vi "Measure distance v2.vi"(8 "error in (no error)":errorcluster, 11 "Input image":T3=refnum) -> (0 "error out":errorcluster)   [LabVIEW 2020]
uses:
  <vilib>/vision/Image Controls.llb/IMAQ Image.ctl
  OOP/MulColLBTable/Object operations.ctl
  Globals/Event FGV Actions.ctl
  TypeDefs/data and image buffer fgv actions.ctl
  <vilib>/Utility/error.llb/whitespace.ctl
  <vilib>/vision/NI_Vision_Development_Module.lvlib
  OOP/MulColLBTable/MulColLBTable-Array/MulColLBTable-Array.lvclass
panel:
  in  "Tab Control":T1(tab)
  in  "Distinct Colours":bool
  in  "Overlay Selected":bool
  in  "Overlay All":bool
  in  "Remove Selected":bool
  in  "Image buffer - Imaging Parameters":i32[](listbox)
  in  "Image buffer - Calibration Parameters":i32[](listbox)
  out "Array 2":dbl[](array[numeric])
  out "min value":dbl
  out "Array":cdb[](array[numeric])
  out "Coordinates":i32[](array[numeric])
  out "Distances":dbl[][](array[numeric])
  out "error out 5":errorcluster
  out "error out 3":errorcluster
  out "error out 7":errorcluster
  out "error out 6":errorcluster
  out "error out 4":errorcluster
  out "Last Mouse Position:All Elements":cluster{"X":i32, "Y":i32}
  out "Circles Data":T2(array[cluster])
  in  "Min Radius":sgl=3.0
  in  "Max Radius":sgl=100.0
  in  "Number of iterations (1)":i32=1
  out "Minimal Value":sgl
  out "Maximal Value":sgl
  out "Image Pixels (U8)":u8[][](array[numeric])
  out "Image size changed":bool
  out "error out 8":errorcluster
  out "error out 9":errorcluster
  out "error out 11":errorcluster
  out "error out 10":errorcluster
  out "Distances 2":sgl[](array[numeric]) format="%.4f"
  in  "Clear Images":bool
  in  "Clear Measurements":bool
  in  "Measurement Mode":T4(ring)
  in  "Re-instate":bool
  out "output cluster":T5 {"Y" format="%.2f"; "X" format="%.2f"}
  out "Image Pixels (I16) 2":i16[][](array[numeric])
  in  "Tab Control 2":enum32{"Grayscale", "Binary", "Intensity"}(tab)
  in  "All":bool
  out "Output Image":T3(plugin-control)
  in  "Grid":bool
  in  "Grid Lines":u32=2 min=1 max=100 step=1
  in  "Image Selector":i32(c297)=7
  out "Output Image 2":T3(plugin-control)
  out "Intensity Graph":i16[][](graph)
  in  "Operation":T6(ring)
  in  "Vertical Pointer Slide":cluster{"Numeric":dbl, "Numeric":dbl}(slide)={"Numeric"=0.0, "Numeric"=254.0} scale=0.0..4096.0
  in  "stop":bool
  # "X Start"
  # "Y start"
  # "X Stop"
  # "X Dist"
  # "Dist"
  # "Y Stop"
  # "Y Dist"
  # "PROTOTYPE ONLY"
  # "This utility is under development, please report any \nissues to the contact details provided on github"
  # "Note : Closing the VI using the top right window close ('X') will only close the front panel - VI keeps running.\nTo completely close this window click 'FINISH/EXIT'"
  # "Current Image data"
  # "Image Processing routines"
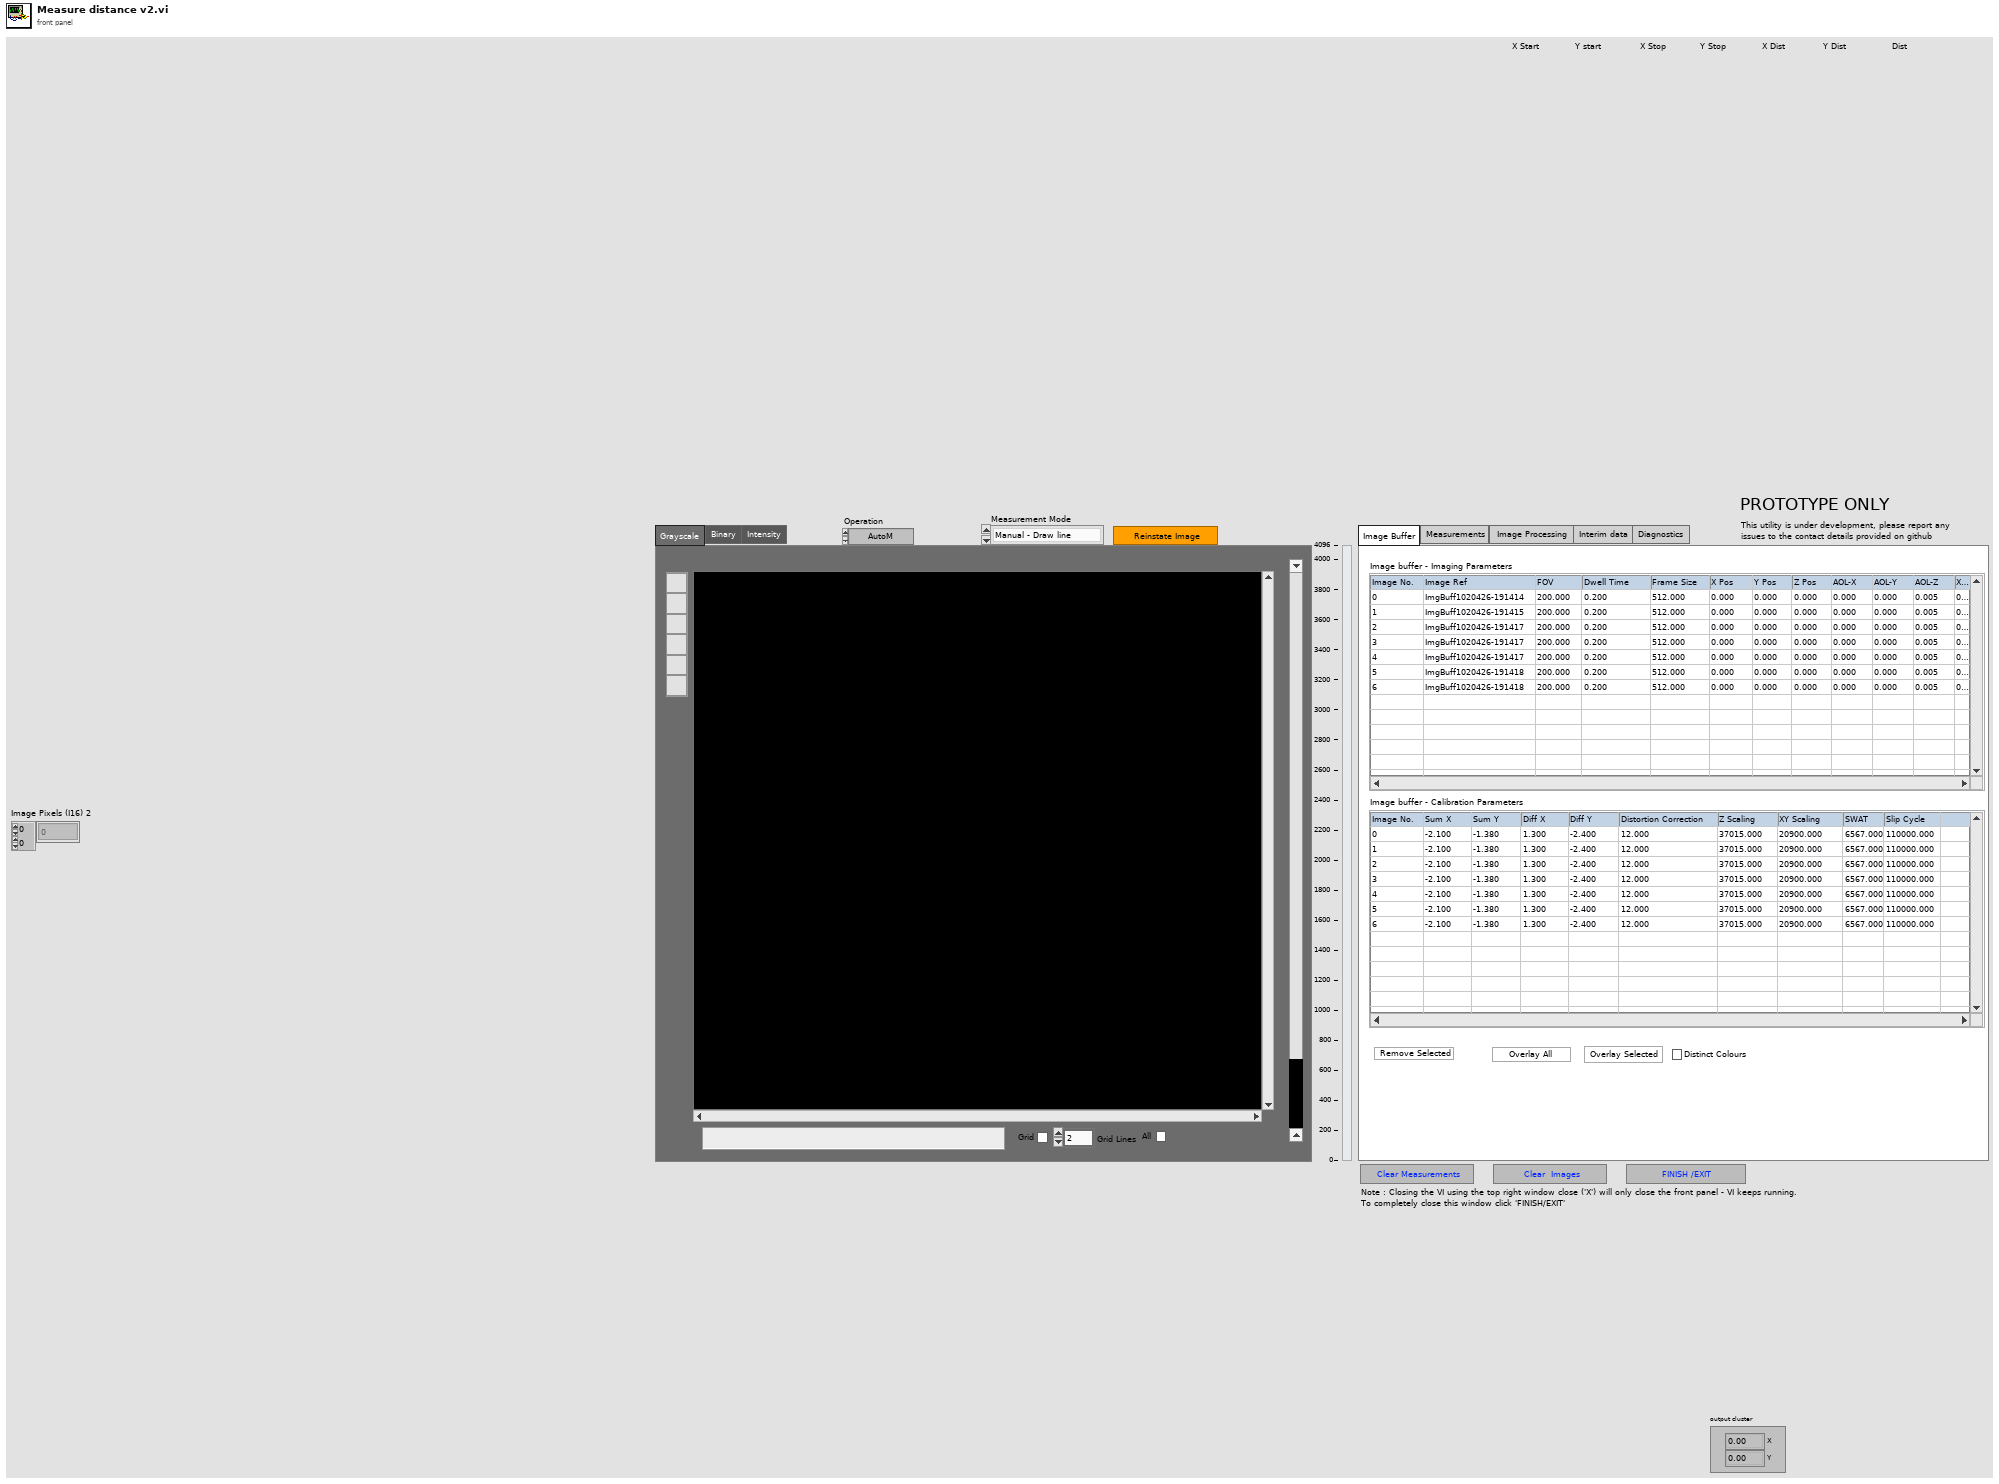
[diagram p1: front panel]
types:
  T1 = enum32{"Image Buffer", "Measurements", "Image Processing  ", "Interim data", "Diagnostics"}
  T2 = cluster{"Pos. X":i32, "Pos. Y":i32, "Radius":i32, "Core Area":i32}[]
  T3 = typedef "IMAQ Image.ctl" = refnum<image>
  T4 = enum16{"Manual - Draw line", "Manual - Circles", "Manual - Points", "Automatic - Circles", "Automatic - Points"}
  T5 = typedef "IMAQ Point" = cluster{"X":sgl, "Y":sgl}
  T6 = enum32{"AutoM", "Close", "Dilate", "Erode", "Gradient", "Gradient out", "Gradient in", "Hit miss", "Open", "PClose", "POpen", "Thick", "Thin"}
  T7 = typedef "Event FGV Actions.ctl" = enum16{"Register Event", "Fire Event", "Release Event"}
  T8 = typedef "Object operations.ctl" = enum16{"Initialise", "Add column headers", "Add rows - bulk", "Stack row - single", "Stack row - multi", "Select row(s)", "Delete row(s)", "Destroy"}
  T9 = typedef "ROI Descriptor" = cluster{"Global Rectangle":i32[], "Contours":cluster{"ID":enum32{"External", "Internal"}, "Type":u32, "Coordinates":i32[]}[]}
  T10 = typedef "data and image buffer fgv actions.ctl" = enum16{"Initialise", "Add Image to buffer", "Read Image buffer", "Edit specific data", "Delete selected image", "Clear all images"}
  T11 = typedef "IMAQ Circle" = cluster{"Center X":i32, "Center Y":i32, "Inner Radius":i32, "Outer Radius":i32, "Start Angle":dbl, "End Angle":dbl}
  T12 = typedef "Current Imaging Parameters.ctl" = cluster{"FOV":dbl, "Dwell Time":dbl, "Frame Size":dbl, "XPos":dbl, "YPos":dbl, "ZPos":dbl, "AOL-X":dbl, "AOL-Y":dbl, "AOL-Z":dbl, "X-Angle":dbl, "Y-Angle":dbl, "Z-Angle":dbl}
  T13 = typedef "Current Calibration Parameters.ctl" = cluster{"Sum X":dbl, "Sum Y":dbl, "Diff X":dbl, "Diff Y":dbl, "Distortion Correction":dbl, "Z_norm to um_scaling":dbl, "X_norm to um_scaling":dbl, "Samples to Wait after Trigger":dbl, "Slip Cycle":dbl}
  T14 = typedef "Image Type" = u32
  T15 = cluster{"histogram":u32[], "Minimal Value":sgl, "Maximal Value":sgl, "Starting Value":sgl, "Interval Width":sgl, "Mean Value":sgl, "Standard  Variation":sgl, "Area (pixels)":i32}
  T16 = typedef "IMAQ Line" = cluster{"Start X":i32, "Start Y":i32, "End X":i32, "End Y":i32}
  T17 = cluster{"Pos. X":i32, "Pos. Y":i32, "Radius":i32, "Core Area":i32}
  T18 = typedef "whitespace.ctl" = u16
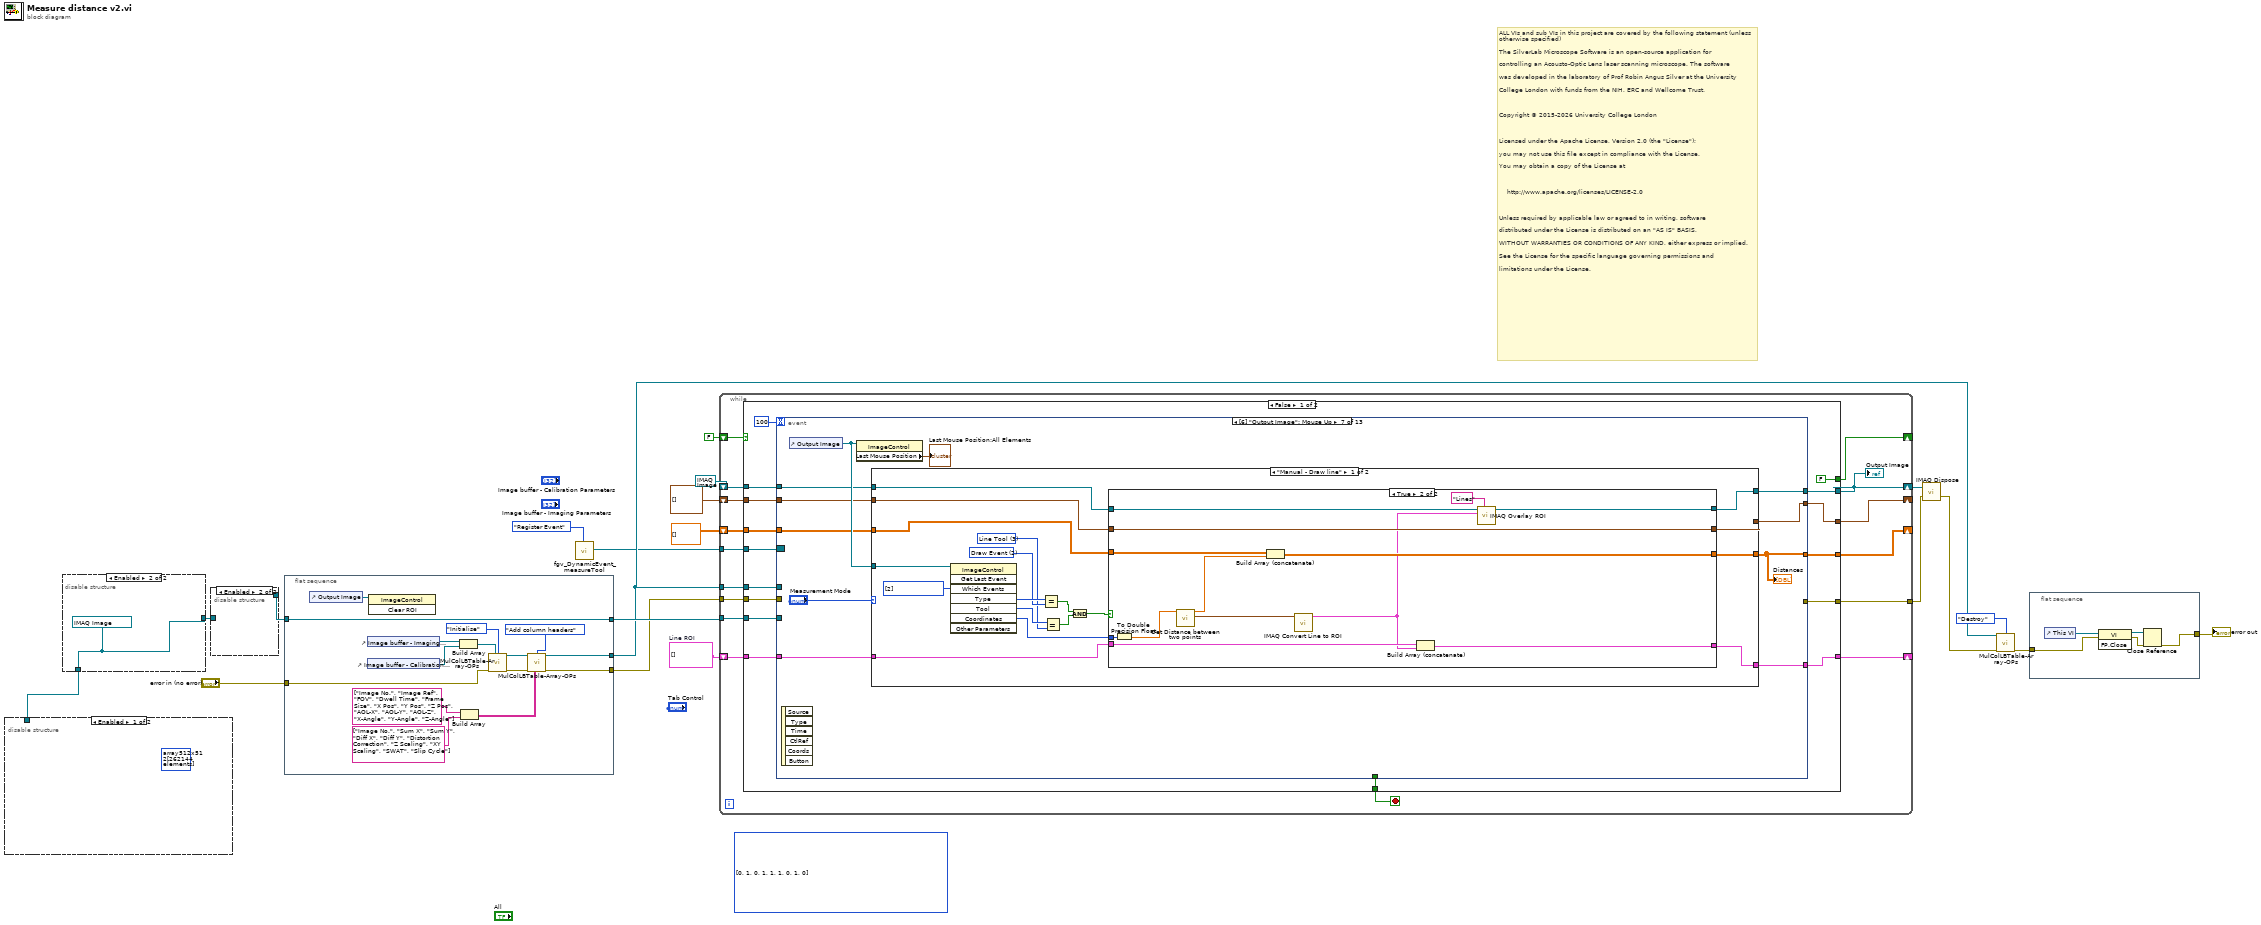
[diagram p0: block diagram]
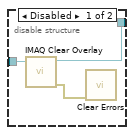
[diagram p2: hidden frame]
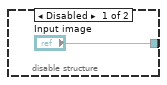
[diagram p3: hidden frame]
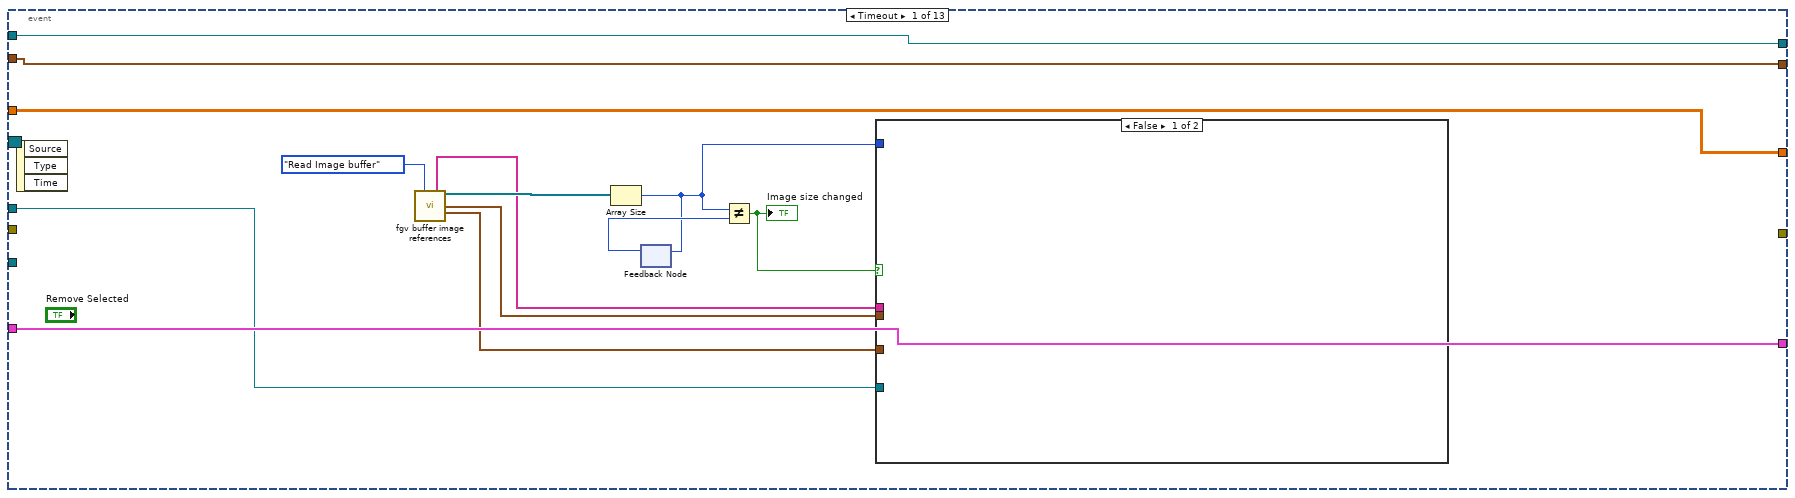
[diagram p5: hidden frame]
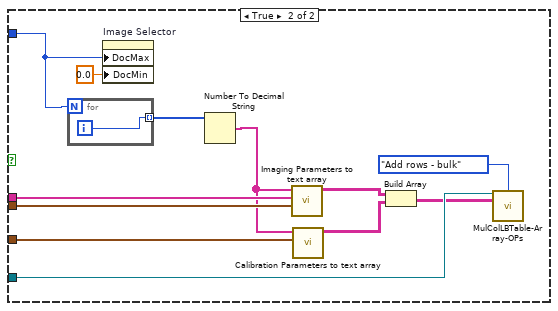
[diagram p6: hidden frame]
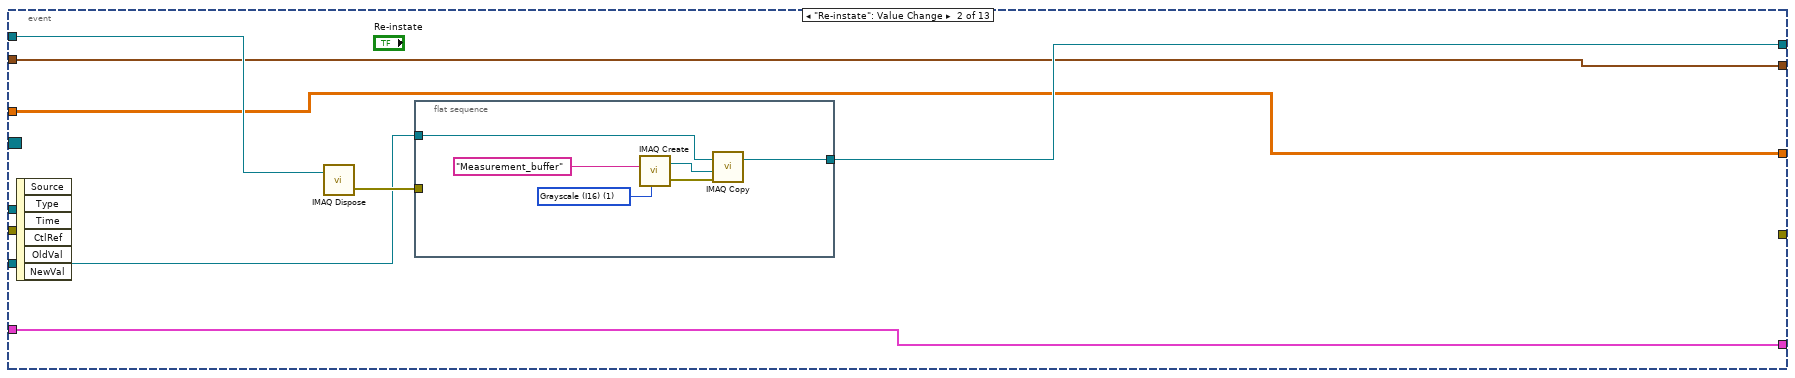
[diagram p7: hidden frame]
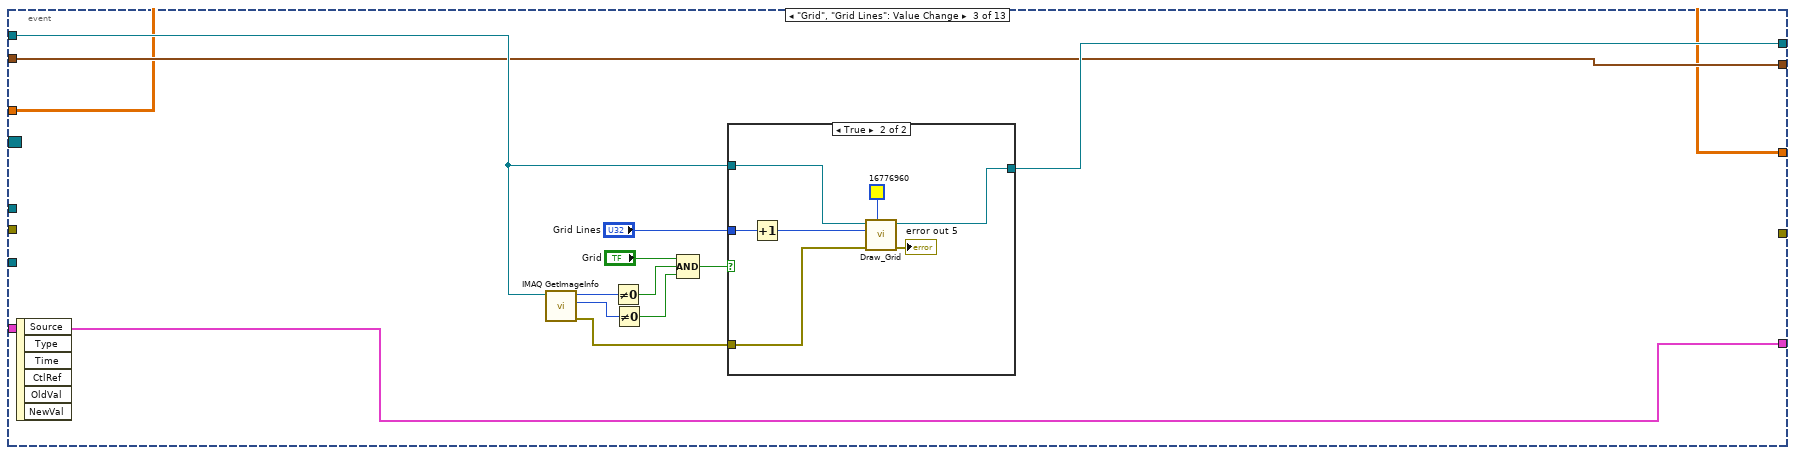
[diagram p8: hidden frame]
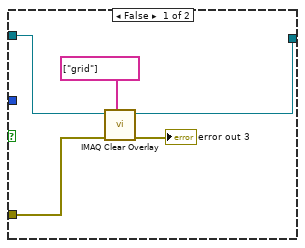
[diagram p9: hidden frame]
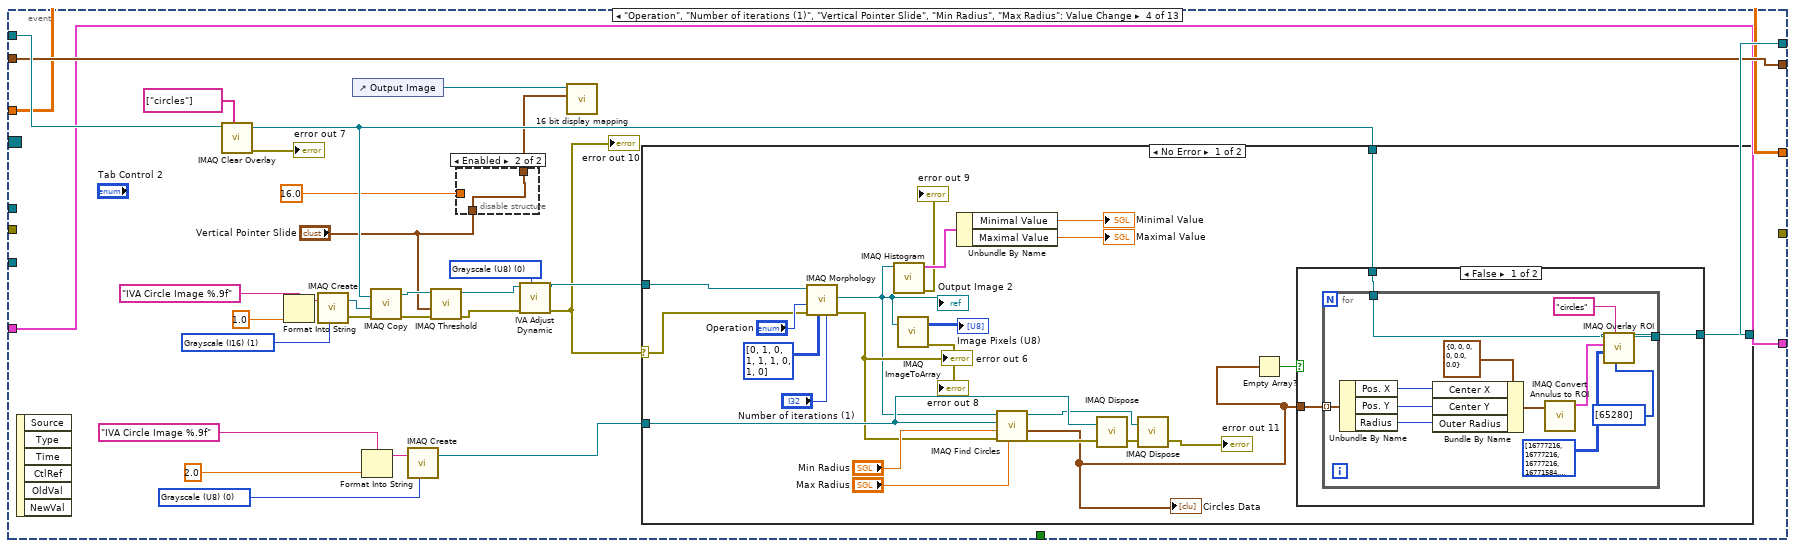
[diagram p10: hidden frame]
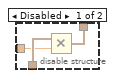
[diagram p11: hidden frame]
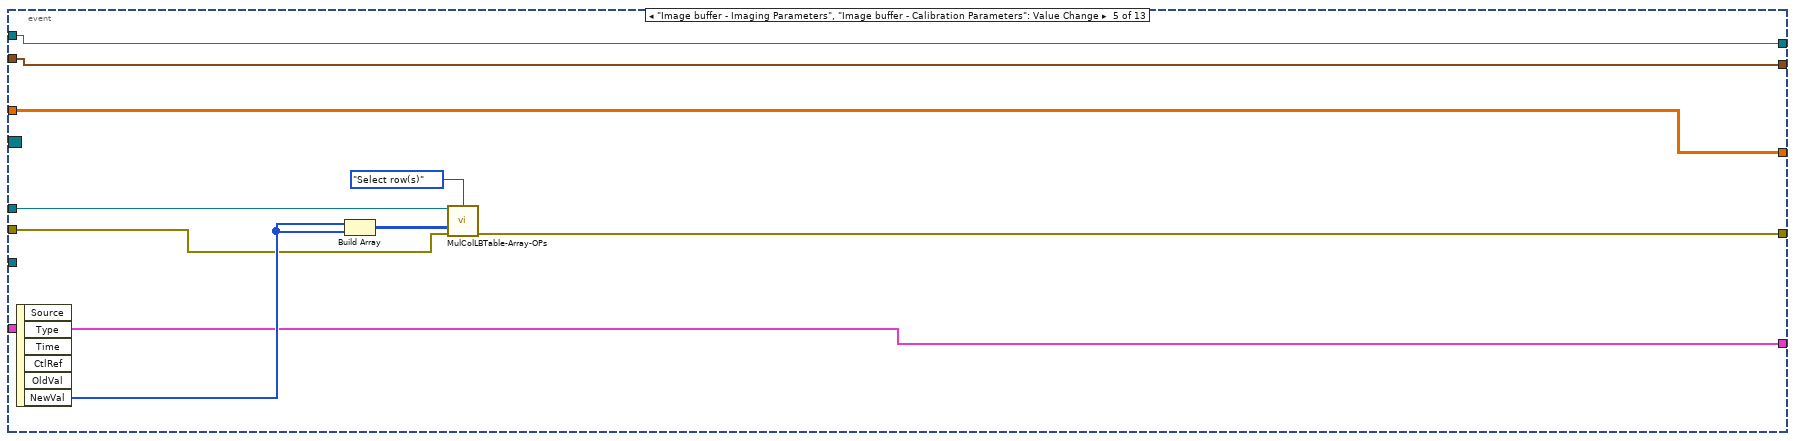
[diagram p14: hidden frame]
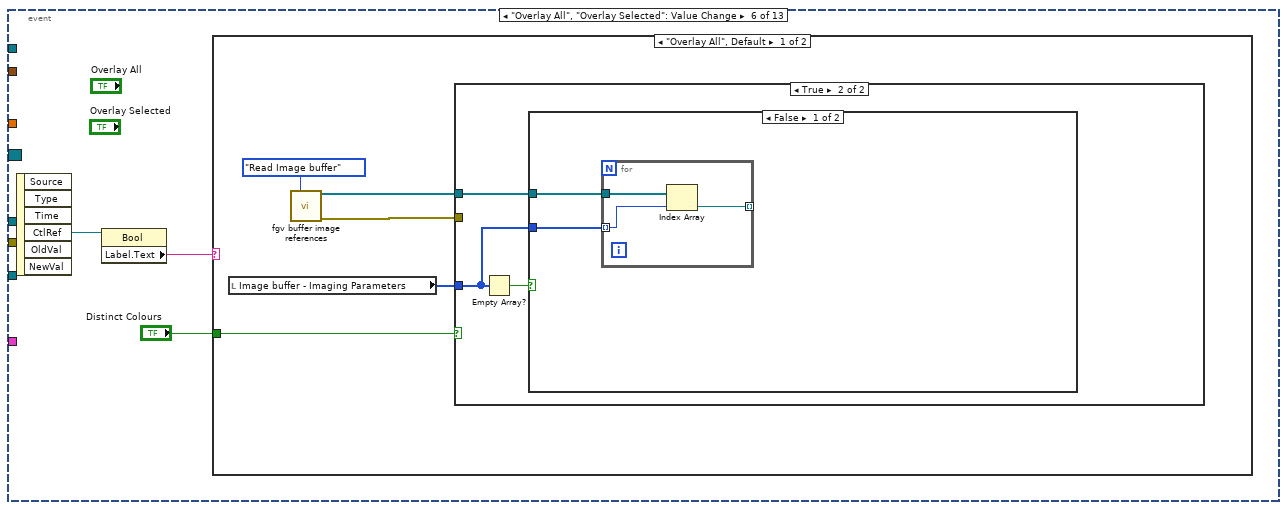
[diagram p15: hidden frame]
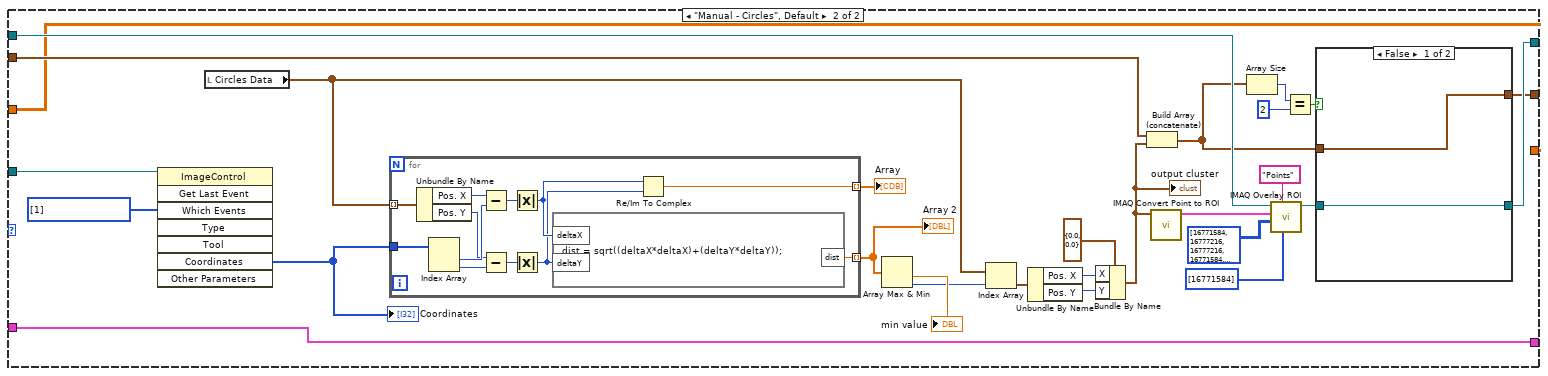
[diagram p20: hidden frame]
diagram:
  w15 = T9[] []  # Line ROI
  (unwired) i32[][] [[0, 1, 0], [1, 1, 1], [0, 1, 0]] ("Structuring Element (Basic Morphology 1) 2")
  # "ALL VIs and sub VIs in this project are covered by the following statement (unless \notherwise specified)\n\nThe SilverLab Microscope Software is an open-source application for\n\ncontrolling an Acousto-Optic Lens laser scanning microscope. The software\n\nwas developed in the laboratory of Prof Robin Angus Silver at the University\n\nCollege London with funds from the NIH, ERC and Wellcome Trust.\n\n \n\nCopyright © 2015-2026 University College London\n\n \n\nLicensed under the Apache License, Version 2.0 (the \"License\");\n\nyou may not use this file except in compliance with the License.\n\nYou may obtain a copy of the License at\n\n \n\n    http://www.apache.org/licenses/LICENSE-2.0\n\n \n\nUnless required by applicable law or agreed to in writing, software\n\ndistributed under the License is distributed on an \"AS IS\" BASIS,\n\nWITHOUT WARRANTIES OR CONDITIONS OF ANY KIND, either express or implied.\n\nSee the License for the specific language governing permissions and\n\nlimitations under the License."
  n1 = disable-structure shown="Enabled" {
    disable-tunnel: ["Input image" w22] -> w14
    disable-tunnel: [_ w22] -> w18
    frame Disabled {
    }
    frame Enabled {
      w22 = T3 refnum ("Input image 2")
    }
  }
  n2 = disable-structure shown="Enabled" {
    disable-tunnel: w18 -> [_ _]
    frame Enabled {
      (unwired) i16[][] array512x512[262144 elements] ("Image Pixels (I16) 2")
    }
    frame Disabled {
    }
  }
  n3 = disable-structure shown="Enabled" {
    disable-tunnel: w14 -> [w25 _]
    disable-tunnel: [w23 _] -> w13
    frame Disabled {
      n4 = call "IMAQ Clear Overlay"("Image"=w25) -> ("error out"=w24:errorcluster, "Image Out"=w23:T3)  [unwired: 9 in]
      n5 = call <vilib>:"Clear Errors.vi"("error in (no error)"=w24) -> ()  [unwired: 5 in, 2 out]
    }
    frame Enabled {
    }
  }
  n6 = flat-sequence {
    tunnel: w13 -> [w39]
    tunnel: [w39] -> w12
    tunnel: [w28] -> w9
    tunnel: [w27] -> w10
    tunnel: "error in (no error)" -> [w26]
    frame #0 {
      n7 = control-ref of="Output Image"() -> (w40:refnum<vi>)
      n8 = control-ref of="Image buffer - Imaging Parameters"() -> (w37:refnum<vi>)
      n9 = control-ref of="Image buffer - Calibration Parameters"() -> (w38:refnum<vi>)
      n10 = invoke class="ImageControl" method="Clear ROI"(reference=w40) -> ()  [unwired: 2 in, 3 out]
      n11 = Build Array(w37, w38) -> (w36:refnum<vi>[])
      n12 = Build Array(string[] ["Image No.", "Image Ref", "FOV", "Dwell Time", "Frame Size", "X Pos", "Y Pos", "Z Pos", "AOL-X", "AOL-Y", "AOL-Z", "X-Angle", "Y-Angle", "Z-Angle"] ("Column Header Strings[]"), string[] ["Image No.", "Sum X", "Sum Y", "Diff X", "Diff Y", "Distortion Correction", "Z Scaling", "XY Scaling", "SWAT", "Slip Cycle"] ("Column Header Strings[]")) -> (w29:string[][])
      n13 = call "MulColLBTable-Array-OPs.vi"("Multi-col LB Refs"=w36, "Operations"=Object_operations."Initialise", "error in (no error)"=w26) -> ("MulColLBTable-Array.lvclass OUT"=w33:refnum<class "MulColLBTable-Array.lvclass">, "error out"=w34:errorcluster)  [unwired: 11 in]
      n14 = call "MulColLBTable-Array-OPs.vi"("MulColLBTable-Array.lvclass IN"=w33, "Operations"=Object_operations."Add column headers", "error in (no error)"=w34, "Column Header Strings[]"=w29) -> ("MulColLBTable-Array.lvclass OUT"=w28:refnum<class "MulColLBTable-Array.lvclass">, "error out"=w27:errorcluster)  [unwired: 10 in]
    }
  }
  n15 = call "fgv_DynamicEvent_measureTool.vi"("Event FGV Actions"=Event_FGV_Actions."Register Event") -> ("Event Registration Refnum"=w3:refnum<event-registration>)  [unwired: 8 in, 2 out]
  n16 = while {
    shift-right: [w52] -> _
    shift-left: FALSE -> [w56]
    tunnel: w12 -> [w55]
    shift-right: [w51] -> w17
    shift-left: T3 refnum ("Image Dst Out") -> [w54]
    shift-right: [w49] -> _
    shift-left: T5[] [] -> [w50]
    shift-right: [w47] -> _
    shift-left: dbl[][] [] ("Distances 2") -> [w48]
    shift-right: [w45] -> _
    shift-left: w15 -> [w46]
    tunnel: w9 -> [w44]
    tunnel: w10 -> [w43]
    tunnel: [w42] -> w5
    tunnel: w3 -> [w41]
    stop <- w53 stop-if-true
    n17 = case shown="False" w56 {
      tunnel: w55 -> [w65 w384]
      tunnel: [w71 w382] -> w51
      tunnel: w54 -> [w72 _]
      tunnel: [w69 FALSE] -> w53
      tunnel: [FALSE FALSE] -> w52
      tunnel: w50 -> [w67 w381]
      tunnel: [w66 w381] -> w49
      tunnel: w48 -> [w64 w379]
      tunnel: [w63 w379] -> w47
      tunnel: w46 -> [w62 w378]
      tunnel: [w61 w378] -> w45
      tunnel: w44 -> [w60 _]
      tunnel: w43 -> [w59 _]
      tunnel: [w58 _] -> w42
      tunnel: w41 -> [w57 _]
      frame False {
        n18 = event shown="[6] \"Output Image\": Mouse Up" {
          selector: w57 -> [_ _ _ _ _ _ _ _ _ _ _ _ _]
          dyn-events: _ -> [_ _ _ _ _ _ _ _ _ _ _ _ _]
          timeout: 100 -> [_ _ _ _ _ _ _ _ _ _ _ _ _]
          tunnel: w72 -> [w85 w105 w123 w152 w216 _ w246 w338 w346 _ _ w364 w375]
          tunnel: [w85 w102 w124 w154 w216 _ w245 w336 w346 w348 _ w364 w375] -> w71
          tunnel: [_ _ _ _ _ _ _ _ _ _ FALSE TRUE w366] -> w69
          tunnel: w67 -> [w84 w101 w114 w149 w215 _ w243 w339 w345 w356 _ w363 w374]
          tunnel: [w84 w101 w114 w149 w215 _ w244 w339 w345 w356 _ w363 w374] -> w66
          tunnel: w65 -> [_ w103 _ _ _ _ _ _ _ _ _ _ _]
          tunnel: w64 -> [w83 w99 w113 w145 w214 _ w241 _ w344 w355 _ w362 w373]
          tunnel: [w83 w99 w113 w145 w214 _ w238 w341 w344 w355 _ w362 w373] -> w63
          tunnel: w62 -> [w82 w100 w112 w144 w212 _ w240 _ w343 w354 _ w361 w372]
          tunnel: [w82 w100 w112 w144 w212 _ w239 w340 w343 w354 _ w361 w372] -> w61
          tunnel: w60 -> [w74 _ _ _ w221 _ _ _ _ _ _ _ _]
          tunnel: w59 -> [_ _ _ _ w217 _ _ _ _ _ _ _ _]
          tunnel: [_ _ _ _ w213 _ _ _ _ _ _ _ _] -> w58
          event Timeout {
            n19 = event-data() -> ()  [unwired: 1 in, 3 out]
            n20 = call "fgv buffer image references.vi"("Actions"=data_and_image_buffer_fgv_actions."Read Image buffer") -> ("Imag ref. name"=w75:string[], "Image Array"=w76:T3[], "Imaging Parameters"=w78:T12[], "Calibration Parameters"=w77:T13[])  [unwired: 8 in, 3 out]
            n21 = Array Size(array=w76) -> (size(s)=w79:i32)
            n22 = feedback-in #1(w79) -> ()
            n23 = feedback #1() -> (w81:i32)  [unwired: 1 in]
            n24 = Not Equal?(x=w79, y=w81) -> (x != y?=w80:bool)
            "Image size changed" <- w80
            n25 = case shown="False" w80 {
              tunnel: w79 -> [_ w95]
              tunnel: w78 -> [_ w93]
              tunnel: w77 -> [_ w91]
              tunnel: w75 -> [_ w94]
              tunnel: w74 -> [_ w88]
              frame False {
              }
              frame True {
                n26 = for {
                  N: w95 -> [_]
                  tunnel: [w98] -> w96 mode=indexing
                  i -> [w98]
                }
                n27 = property on="Image Selector" class="Scroll (strict)"("DocMax"=w95, "DocMin"=0.0 ("Doc Min")) -> ()  [unwired: 2 in, 2 out]
                n28 = Number To Decimal String(number=w96) -> (decimal integer string=w92:string[])  [unwired: 1 in]
                n29 = call "Imaging Parameters to text array.vi"("Imaging Parameters"=w93, "Image Ref"=w94, "Image No"=w92) -> ("Imaging Parameters"=w90:string[][])  [unwired: 8 in]
                n30 = call "Calibration Parameters to text array.vi"("Calibration Parameters"=w91, "Image No"=w92) -> ("Calibration Parameters"=w89:string[][])  [unwired: 9 in]
                n31 = Build Array(w90, w89) -> (w86:string[][][])
                n32 = call "MulColLBTable-Array-OPs.vi"("MulColLBTable-Array.lvclass IN"=w88, "Operations"=Object_operations."Add rows - bulk", "Item Names - Bulk / stack Multiple"=w86) -> ()  [unwired: 11 in, 2 out]
              }
            }
          }
          event "Re-instate": Value Change {
            n33 = event-data() -> ()  [unwired: 1 in, 6 out]
            n34 = call "IMAQ Dispose"("Image"=w105) -> ("error out"=w104:errorcluster)  [unwired: 5 in]
            n35 = flat-sequence {
              tunnel: w104 -> [_]
              tunnel: w103 -> [w107]
              tunnel: [w106] -> w102
              frame #0 {
                w108 = T14 1 items=["Grayscale (U8)", "Grayscale (I16)", "Grayscale (SGL)", "Complex (CSG)", "RGB (U32)", "HSL (U32)", "RGB (U64)", "Grayscale (U16)"] ("Image Type")
                n36 = call "IMAQ Create"("Image Name"="Measurement_buffer", "Image Type"=w108) -> ("New Image"=w110:T3, "error out"=w111:errorcluster)  [unwired: 3 in]
                n37 = call "IMAQ Copy"("error in (no error)"=w111, "Image Dst"=w110, "Image Src"=w107) -> ("Image Dst Out"=w106:T3)  [unwired: 3 in, 1 out]
              }
            }
          }
          event "Grid", "Grid Lines": Value Change {
            n38 = event-data() -> ()  [unwired: 1 in, 6 out]
            n39 = call "IMAQ GetImageInfo"("Image"=w123) -> ("error out"=w117:errorcluster, "Y Resolution"=w120:i32, "X Resolution"=w121:i32)  [unwired: 3 in, 5 out]
            n40 = Not Equal To 0?(x=w121) -> (x != 0?=w119:bool)
            n41 = Not Equal To 0?(x=w120) -> (x != 0?=w118:bool)
            n42 = Compound Arithmetic op=AND("Grid", w119, w118) -> (w116:bool)
            n43 = case shown="True" w116 {
              tunnel: w123 -> [w128 w136]
              tunnel: [w127 w135] -> w124
              tunnel: w117 -> [w125 w133]
              tunnel: "Grid Lines" -> [_ w131]
              frame False {
                n44 = call "IMAQ Clear Overlay"("Groups"=string[] ["grid"], "error in (no error)"=w125, "Image"=w128) -> ("error out"=→"error out 3":errorcluster, "Image Out"=w127:T3)  [unwired: 7 in]
              }
              frame True {
                n45 = Increment(x=w131) -> (x+1=w130:u32)
                n46 = call "Draw_Grid.vi"("Grid Line Color"=u32 16776960, "error in (no error)"=w133, "Grid Lines"=w130, "Image In"=w136) -> ("error out"=→"error out 5":errorcluster, "Image Out"=w135:T3)  [unwired: 6 in]
              }
            }
          }
          event "Operation", "Number of iterations (1)", "Vertical Pointer Slide", "Min Radius", "Max Radius": Value Change {
            w158 = T14 0 items=["Grayscale (U8)", "Grayscale (I16)", "Grayscale (SGL)", "Complex (CSG)", "RGB (U32)", "HSL (U32)", "RGB (U64)", "Grayscale (U16)"] ("Image Type")
            w159 = T14 0 items=["Grayscale (U8)", "Grayscale (I16)", "Grayscale (SGL)", "Complex (CSG)", "RGB (U32)", "HSL (U32)", "RGB (U64)", "Grayscale (U16)"] ("Image Type")
            w164 = T14 1 items=["Grayscale (U8)", "Grayscale (I16)", "Grayscale (SGL)", "Complex (CSG)", "RGB (U32)", "HSL (U32)", "RGB (U64)", "Grayscale (U16)"] ("Image Type")
            n47 = event-data() -> ()  [unwired: 1 in, 6 out]
            n48 = call "IMAQ Clear Overlay"("Groups"=string[] ["circles"], "Image"=w152) -> ("error out"=→"error out 7":errorcluster, "Image Out"=w151:T3)  [unwired: 8 in]
            n49 = Format Into String(format string="IVA Circle Image %.9f" ("Image Name"), 1.0) -> (resulting string=w166:string)  [unwired: 2 in, 1 out]
            n50 = call "IMAQ Create"("Image Name"=w166, "Image Type"=w164) -> ("New Image"=w156:T3, "error out"=w157:errorcluster)  [unwired: 2 in, 1 out]
            n51 = control-ref of="Output Image"() -> (w148:refnum<vi>)
            n52 = Format Into String(format string="IVA Circle Image %.9f" ("Image Name"), 2.0) -> (resulting string=w162:string)  [unwired: 2 in, 1 out]
            n53 = call "IMAQ Copy"("error in (no error)"=w157, "Image Dst"=w156, "Image Src"=w151) -> ("error out"=w142:errorcluster, "Image Dst Out"=w143:T3)  [unwired: 3 in]
            n54 = call "IMAQ Create"("Image Name"=w162, "Image Type"=w159) -> ("New Image"=w155:T3)  [unwired: 2 in, 2 out]
            n55 = call "IMAQ Threshold"("error in (no error)"=w142, "Range"="Vertical Pointer Slide", "Image Src"=w143) -> ("error out"=w141:errorcluster, "Image Dst Out"=w140:T3)  [unwired: 3 in, 4 out]
            n56 = disable-structure shown="Enabled" {
              disable-tunnel: "Vertical Pointer Slide" -> [w169 w170]
              disable-tunnel: 16.0 -> [w168 _]
              disable-tunnel: [w167 w170] -> w146
              frame Disabled {
                n57 = Multiply(x=w169, y=w168) -> (x*y=w167:cluster{"Numeric":dbl, "Numeric":dbl})
              }
              frame Enabled {
              }
            }
            n58 = call <vilib>:"IVA Adjust Dynamic.vi"("Image Type"=w158, "error in (no error)"=w141, "Image Src"=w140) -> ("error out"=w138:errorcluster, "Image Out"=w139:T3)  [unwired: 7 out]
            "error out 10" <- w138
            n59 = call "16 bit display mapping.vi"("16 bit display mapping"=w146, "Image Display"=w148) -> ()  [unwired: 8 in, 2 out]
            n60 = case shown="No Error" w138 {
              selector: w138 -> [w171 _]
              tunnel: w155 -> [w189 w211]
              tunnel: [w186 w211] -> w154
              tunnel: w139 -> [w172 _]
              tunnel: w151 -> [w184 _]
              frame No Error {
                n61 = call "IMAQ Morphology"("Number of iterations (1)"="Number of iterations (1)", "Structuring Element"=i32[][] [[0, 1, 0], [1, 1, 1], [0, 1, 0]] ("Structuring Element (Basic Morphology 1) 2"), "error in (no error)"=w171, "Operation"="Operation", "Image Src"=w172) -> ("error out"=w180:errorcluster, "Image Dst Out"=w178:T3)  [unwired: 2 in, 3 out]
                "error out 6" <- w180
                "Output Image 2" <- w178
                n62 = call "IMAQ Histogram"("Image"=w178) -> ("error out"=→"error out 9":errorcluster, "Histogram Report"=w183:T15)  [unwired: 4 in, 5 out]
                n63 = call "IMAQ ImageToArray"("Image"=w178) -> ("error out"=→"error out 8":errorcluster, "Image Pixels (U8)"=→"Image Pixels (U8)":u8[][])  [unwired: 3 in, 3 out]
                n64 = Unbundle By Name(w183) -> ("Minimal Value"=→"Minimal Value":sgl, "Maximal Value"=→"Maximal Value":sgl)
                n65 = call "IMAQ Find Circles"("Max Radius"="Max Radius", "error in (no error)"=w180, "Min Radius"="Min Radius", "Image Dst"=w189, "Image Src"=w178) -> ("error out"=w190:errorcluster, "Circles Data"=w174:T2, "Image Dst Out"=w187:T3)  [unwired: 4 out]
                "Circles Data" <- w174
                n66 = call "IMAQ Dispose"("Image"=w189, "error in (no error)"=w190) -> ("error out"=w188:errorcluster)  [unwired: 1 in, 3 out]
                n67 = call "IMAQ Dispose"("Image"=w187, "error in (no error)"=w188) -> ("error out"=→"error out 11":errorcluster)  [unwired: 1 in, 3 out]
                n68 = Empty Array?(array=w174) -> (empty?=w173:bool)
                n69 = case shown="False" w173 {
                  tunnel: [w197 w210] -> w186
                  tunnel: w184 -> [w196 w210]
                  tunnel: w174 -> [w195 _]
                  frame False {
                    n70 = for {
                      tunnel: w195 -> [w208] mode=indexing
                      tunnel: w196 -> [w203]
                      tunnel: [w199] -> w197
                      n71 = Unbundle By Name(w208) -> ("Pos. X"=w207:i32, "Pos. Y"=w206:i32, "Radius"=w205:i32)
                      n72 = Bundle By Name(cluster=T11 {"Center X"=0, "Center Y"=0, "Inner Radius"=0, "Outer Radius"=0, "Start Angle"=0.0, "End Angle"=0.0} ("Annulus"), "Center X"=w207, "Center Y"=w206, "Outer Radius"=w205) -> (w204:T11)
                      n73 = call "IMAQ Convert Annulus to ROI"("Annulus"=w204) -> ("ROI Descriptor"=w202:T9)  [unwired: 8 in, 1 out]
                      n74 = call "IMAQ Overlay ROI"("Colors (Green)"=u32[] [65280], "Group"="circles", "Point Symbol"=u32[][] [[16777216, 16777216, 16777216, 16771584, 16777216, 16777216, 16777216], [16777216, 16777216, 16777216, 16771584, 16777216, 16777216, 16777216], [16777216, 16777216, 16777216, 16771584, 16777216, 16777216, 16777216], [16771584, 16771584, 16771584, 16771584, 16771584, 16771584, 16771584], [16777216, 16777216, 16777216, 16771584, 16777216, 16777216, 16777216], [16777216, 16777216, 16777216, 16771584, 16777216, 16777216, 16777216], [16777216, 16777216, 16777216, 16771584, 16777216, 16777216, 16777216]], "ROI Descriptor"=w202, "Image"=w203) -> ("Image Out"=w199:T3)  [unwired: 5 in, 1 out]
                    }
                  }
                  frame True {
                  }
                }
              }
              frame Error {
              }
            }
          }
          event "Image buffer - Imaging Parameters", "Image buffer - Calibration Parameters": Value Change {
            n75 = event-data() -> ("NewVal"=w219:i32[])  [unwired: 1 in, 5 out]
            n76 = Build Array(w219, w219) -> (w218:i32[][])
            n77 = call "MulColLBTable-Array-OPs.vi"("MulColLBTable-Array.lvclass IN"=w221, "Operations"=Object_operations."Select row(s)", "Value"=w218, "error in (no error)"=w217) -> ("error out"=w213:errorcluster)  [unwired: 10 in, 1 out]
          }
          event "Overlay All", "Overlay Selected": Value Change {
            n78 = event-data() -> ("CtlRef"=w224:refnum<vi>)  [unwired: 1 in, 5 out]
            n79 = property class="Bool"(reference=w224) -> ("Label.Text"=w223:string)  [unwired: 1 in, 2 out]
            n80 = case shown="\"Overlay All\", Default" w223 {
              tunnel: "Distinct Colours" -> [w229 _]
              frame "Overlay All", Default {
                n81 = local read "Image buffer - Imaging Parameters"() -> (w226:i32[])
                n82 = call "fgv buffer image references.vi"("Actions"=data_and_image_buffer_fgv_actions."Read Image buffer") -> ("Image Array"=w227:T3[], "error out"=w228:errorcluster)  [unwired: 8 in, 5 out]
                n83 = case shown="True" w229 {
                  tunnel: w228 -> [_ _]
                  tunnel: w227 -> [_ w232]
                  tunnel: w226 -> [_ w230]
                  frame False {
                  }
                  frame True {
                    n84 = Empty Array?(array=w230) -> (empty?=w231:bool)
                    n85 = case shown="False" w231 {
                      tunnel: w232 -> [w234 _]
                      tunnel: w230 -> [w233 _]
                      frame False {
                        n86 = for {
                          tunnel: w234 -> [w237]
                          tunnel: w233 -> [w236] mode=indexing
                          tunnel: [w235] -> _ mode=indexing
                          n87 = Index Array(array=w237, index=w236) -> (element=w235:T3)
                        }
                      }
                      frame True {
                      }
                    }
                  }
                }
              }
              frame "Overlay Selected" {
              }
            }
          }
          event "Output Image": Mouse Up {
            n88 = event-data() -> ()  [unwired: 1 in, 6 out]
            n89 = control-ref of="Output Image"() -> (w247:refnum<vi>)
            n90 = property class="ImageControl"(reference=w247) -> ("Last Mouse Position"=→"Last Mouse Position:All Elements":cluster{"X":i32, "Y":i32})  [unwired: 1 in, 2 out]
            n91 = case shown="\"Manual - Draw line\"" "Measurement Mode" {
              tunnel: w247 -> [w265 w311]
              tunnel: w246 -> [w254 w297]
              tunnel: [w253 w291] -> w245
              tunnel: [w252 w290] -> w244
              tunnel: w243 -> [w251 w289]
              tunnel: w241 -> [w256 w285]
              tunnel: [w255 w285] -> w238
              tunnel: w240 -> [w250 w284]
              tunnel: [w249 w284] -> w239
              frame "Manual - Draw line" {
                w261 = 3 items=["None", "Selection Tool", "Point Tool", "Line Tool", "Rectangle Tool", "Oval Tool", "Polygon Tool", "ClosedFreehandTool", "Annulus Tool", "Rotated Rectangle Tool", "Zoom Tool", "Pan Tool", "Polyline Tool", "Freehand Tool"] ("Tool")
                w263 = 2 items=["No Event"=0, "Click Event"=1, "Draw Event"=2, "Size Event"=4, "Scroll Event"=5, "Double Click Event"=8] ("Type 2")
                w266 = i32[] [2] items=["No Event"=0, "Click Event"=1, "Draw Event"=2, "Size Event"=4, "Scroll Event"=5, "Double Click Event"=8] ("Which Events")
                n92 = invoke class="ImageControl" method="Get Last Event"(reference=w265, "Which Events"=w266) -> ("Type"=w264:i32, "Tool"=w262:i32, "Coordinates"=w257:i32[])  [unwired: 6 in, 5 out]
                n93 = Equal?(x=w264, y=w263) -> (x = y?=w260:bool)
                n94 = Equal?(x=w262, y=w261) -> (x = y?=w259:bool)
                n95 = And(x=w260, y=w259) -> (x .and. y?=w258:bool)
                n96 = case shown="True" w258 {
                  tunnel: w257 -> [_ w283]
                  tunnel: w256 -> [w270 w281]
                  tunnel: [w270 w280] -> w255
                  tunnel: w254 -> [w269 w278]
                  tunnel: [w269 w277] -> w253
                  tunnel: [w268 w276] -> w252
                  tunnel: w251 -> [w268 w276]
                  tunnel: w250 -> [w267 w275]
                  tunnel: [w267 w274] -> w249
                  frame False {
                  }
                  frame True {
                    n97 = To Double Precision Float(number=w283) -> (double precision float=w282:dbl[])
                    n98 = call "Get Distance between two points.vi"("Array"=w282) -> ("Line ROI coordinates"=w271:T16, "appended array"=w279:dbl[])  [unwired: 9 in]
                    n99 = Build Array (concatenate)(w281, w279) -> (w280:dbl[][])
                    n100 = call "IMAQ Convert Line to ROI"("Line"=w271) -> ("ROI Descriptor"=w273:T9)  [unwired: 8 in, 1 out]
                    n101 = Build Array (concatenate)(w275, w273) -> (w274:T9[])
                    n102 = call "IMAQ Overlay ROI"("Group"="Lines", "ROI Descriptor"=w273, "Image"=w278) -> ("Image Out"=w277:T3)  [unwired: 7 in, 1 out]
                  }
                }
              }
              frame "Manual - Circles", Default {
                w286 = i32[] [1] items=["No Event"=0, "Click Event"=1, "Draw Event"=2, "Size Event"=4, "Scroll Event"=5, "Double Click Event"=8] ("Which Events")
                n103 = invoke class="ImageControl" method="Get Last Event"(reference=w311, "Which Events"=w286) -> ("Coordinates"=w307:i32[])  [unwired: 6 in, 7 out]
                "Coordinates" <- w307
                n104 = local read "Circles Data"() -> (w298:T2)
                n105 = for {
                  tunnel: w298 -> [w334] mode=indexing
                  tunnel: w307 -> [w333]
                  tunnel: [w328] -> w309 mode=indexing
                  tunnel: [w327] -> w310 mode=indexing
                  n106 = Unbundle By Name(w334) -> ("Pos. X"=w326:i32, "Pos. Y"=w324:i32)
                  n107 = Index Array(array=w333) -> (element #1=w325:i32, element #2=w323:i32)  [unwired: 2 in]
                  n108 = Subtract(x=w326, y=w325) -> (x-y=w332:i32)
                  n109 = Subtract(x=w324, y=w323) -> (x-y=w331:i32)
                  n110 = Absolute Value(x=w332) -> (abs(x)=w330:i32)
                  n111 = Absolute Value(x=w331) -> (abs(x)=w329:i32)
                  n112 = formula code="dist = sqrt((deltaX*deltaX)+(deltaY*deltaY));"("deltaX"=w330, "deltaY"=w329) -> ("dist"=w328:dbl)
                  n113 = Re/Im To Complex(1:w329, 2:w330) -> (0:w327:cdb)
                }
                "Array" <- w310
                "Array 2" <- w309
                n114 = Array Max & Min(array=w309) -> (min value=→"min value":dbl, min index (indices)=w296:i32)  [unwired: 2 out]
                n115 = Index Array(array=w298, index=w296) -> (element=w306:T17)
                n116 = Unbundle By Name(w306) -> ("Pos. X"=w305:i32, "Pos. Y"=w304:i32)
                n117 = Bundle By Name(cluster=T5 {"X"=0.0, "Y"=0.0} ("Point"), "X"=w305, "Y"=w304) -> (w288:T5)
                "output cluster" <- w288
                n118 = Build Array (concatenate)(w289, w288) -> (w287:T5[])
                n119 = call "IMAQ Convert Point to ROI"("Point"=w288) -> ("ROI Descriptor"=w302:T9)  [unwired: 8 in, 1 out]
                n120 = Array Size(array=w287) -> (size(s)=w295:i32)
                n121 = call "IMAQ Overlay ROI"("Colors (Green)"=u32[] [16771584], "Group"="Points", "Point Symbol"=u32[][] [[16771584, 16777216, 16777216, 16771584, 16777216, 16777216, 16771584], [16777216, 16771584, 16777216, 16771584, 16777216, 16771584, 16777216], [16777216, 16777216, 16771584, 16771584, 16771584, 16777216, 16777216], [16771584, 16771584, 16771584, 16771584, 16771584, 16771584, 16771584], [16777216, 16777216, 16771584, 16771584, 16771584, 16777216, 16777216], [16777216, 16771584, 16777216, 16771584, 16777216, 16771584, 16777216], [16771584, 16777216, 16777216, 16771584, 16777216, 16777216, 16771584]], "ROI Descriptor"=w302, "Image"=w297) -> ("Image Out"=w292:T3)  [unwired: 5 in, 1 out]
                n122 = Equal?(x=w295, y=2) -> (x = y?=w293:bool)
                n123 = case shown="False" w293 {
                  tunnel: w287 -> [w312 w318]
                  tunnel: w292 -> [w313 w321]
                  tunnel: [w313 w320] -> w291
                  tunnel: [w312 T5[] []] -> w290
                  frame False {
                  }
                  frame True {
                    n124 = call "IMAQ Point Distances"("Points"=w318) -> ("Distances"=→"Distances 2":sgl[])  [unwired: 4 in, 1 out]
                    n125 = Index Array(array=w318) -> (element #1=w317:T5, element #2=w316:T5)  [unwired: 2 in]
                    n126 = call "IMAQ Overlay Line"("Color"=u32 16771584, "Group"="Line", "End Point"=w316, "Start Point"=w317, "Image"=w321) -> ("Image Out"=w320:T3)  [unwired: 5 in, 1 out]
                  }
                }
              }
            }
            "Distances" <- w238
          }
          event "Clear Measurements": Value Change {
            w340 = T9[] []  # Line ROI
            w341 = dbl[][] [] ("Distances 2")
            n127 = event-data() -> ()  [unwired: 1 in, 6 out]
            n128 = call "IMAQ Clear Overlay"("Image"=w338) -> ("error out"=w337:errorcluster, "Image Out"=w336:T3)  [unwired: 9 in]
            n129 = control-ref of="Output Image"() -> (w335:refnum<vi>)
            n130 = call <vilib>:"Clear Errors.vi"("error in (no error)"=w337) -> ()  [unwired: 5 in, 2 out]
            n131 = invoke class="ImageControl" method="Clear ROI"(reference=w335) -> ()  [unwired: 2 in, 3 out]
            n132 = local write "Distances"(w341) -> ()
          }
          event "Clear Images": Value Change {
            n133 = event-data() -> ()  [unwired: 1 in, 6 out]
            n134 = call "fgv buffer image references.vi"("Actions"=data_and_image_buffer_fgv_actions."Clear all images") -> ()  [unwired: 8 in, 7 out]
          }
          event "Image Selector": Value Change {
            n135 = event-data() -> ()  [unwired: 1 in, 6 out]
            n136 = call "fgv buffer image references.vi"("Actions"=data_and_image_buffer_fgv_actions."Read Image buffer") -> ("Image Array"=w353:T3[])  [unwired: 8 in, 6 out]
            n137 = Index Array(array=w353, index="Image Selector") -> (element=w348:T3)
            n138 = call "IMAQ ImageToArray"("Image"=w348) -> ("Image Pixels (I16)"=w350:i16[][])  [unwired: 3 in, 4 out]
            "Image Pixels (I16) 2" <- w350
            n139 = Transpose 2D Array(2D array=w350) -> (transposed array=w349:i16[][])
            n140 = for {
              tunnel: w349 -> [w358] mode=indexing
              tunnel: [w357] -> w351 mode=indexing
              n141 = Reverse 1D Array(array=w358) -> (reversed array=w357:i16[])
            }
            "Intensity Graph" <- w351
          }
          event Panel Close {
            n142 = event-data() -> ()  [unwired: 1 in, 4 out]
            n143 = control-ref of="This VI"() -> (w360:refnum<vi>)
            n144 = invoke class="VI" method="FP.Close"(reference=w360) -> ()  [unwired: 2 in, 3 out]
          }
          event "stop": Value Change {
            n145 = event-data() -> ()  [unwired: 1 in, 6 out]
          }
          event User Event {
            w370 = T18 0 items=["both", "start of string", "end of string"] ("location (both)")
            n146 = event-data() -> ("element"=w371:string)  [unwired: 1 in, 4 out]
            n147 = call <vilib>:"Trim Whitespace.vi"("string"=w371, "location (both)"=w370) -> ("trimmed string"=w369:string)
            n148 = Equal?(x=w369, y="stop") -> (x = y?=w367:bool)
            n149 = case shown="True" w367 {
              tunnel: [FALSE TRUE] -> w366
              frame False {
              }
              frame True {
              }
            }
          }
        }
      }
      frame True {
        w388 = T14 1 items=["Grayscale (U8)", "Grayscale (I16)", "Grayscale (SGL)", "Complex (CSG)", "RGB (U32)", "HSL (U32)", "RGB (U64)", "Grayscale (U16)"] ("Image Type")
        n150 = call "IMAQ Create"("Image Name"="Measurement_buffer", "Image Type"=w388) -> ("New Image"=w383:T3, "error out"=w387:errorcluster)  [unwired: 3 in]
        n151 = call "IMAQ Copy"("error in (no error)"=w387, "Image Dst"=w383, "Image Src"=w384) -> ("Image Dst Out"=w382:T3)  [unwired: 3 in, 1 out]
        n152 = local write "Output Image"(w382) -> ()
      }
    }
    "Output Image" <- w51
  }
  n153 = call "IMAQ Dispose"("Image"=w17, "error in (no error)"=w5) -> ("error out"=w7:errorcluster)  [unwired: 4 in]
  n154 = call "MulColLBTable-Array-OPs.vi"("MulColLBTable-Array.lvclass IN"=w9, "Operations"=Object_operations."Destroy", "error in (no error)"=w7) -> ("error out"=w2:errorcluster)  [unwired: 11 in, 1 out]
  n155 = flat-sequence {
    tunnel: w2 -> [w390]
    tunnel: [w389] -> w1
    frame #0 {
      n156 = control-ref of="This VI"() -> (w393:refnum<vi>)
      n157 = invoke class="VI" method="FP.Close"(reference=w393, error in=w390) -> (reference out=w392:refnum<vi>, error out=w391:errorcluster)  [unwired: 1 in, 1 out]
      n158 = Close Reference(reference=w392, error in (no error)=w391) -> (error out=w389:errorcluster)
    }
  }
  "error out" <- w1
